vi "ZTarget.vi"(2 "PID gains for Z angle":T1={"proportional gain (Kc)"=0.03, "integral time (Ti, min)"=0.0, "derivative time (Td, min)"=0.001} {"derivative time (Td, min)" format="%.3f"; "integral time (Ti, min)" format="%.3f"; "proportional gain (Kc)" format="%.3f"}, 3 "Lower Array":dbl[](array[numeric])=[-14.0, 14.0, -59.0, 59.0, -121.0, 121.0, -166.0, 166.0, -180.0], 4 "Upper Array":dbl[](array[numeric])=[14.0, 59.0, -14.0, 121.0, -59.0, 166.0, -121.0, 190.0, -166.0], 5 "Target Values":dbl[](array[numeric])=[0.0, 28.0, -28.0, 90.0, -90.0, 152.0, -152.0, 180.0, 180.0], 6 "Zin":dbl) -> (0 "Z Out":dbl)   [LabVIEW 2018]
uses:
  Robot Global Data.vi
  <vilib>/addons/control/pid/pid.llb/PID (DBL).vi
  <vilib>/addons/control/pid/NI_PID_pid.lvlib
panel:
  out "ZTarget":dbl=180.0 format="%#_13g"
  out "In Range?":bool[](array[boolean])=[FALSE, FALSE, FALSE, FALSE, FALSE, FALSE, FALSE, FALSE, TRUE]
  in  "Auto Z":bool=TRUE
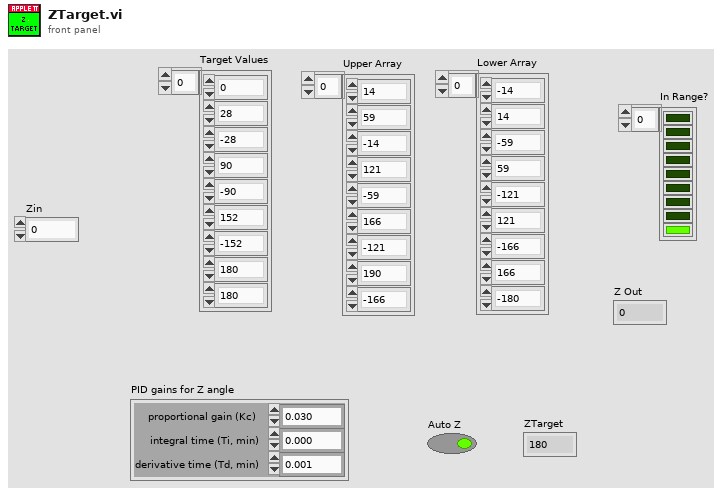
[diagram p1: front panel]
types:
  T1 = cluster{"proportional gain (Kc)":dbl, "integral time (Ti, min)":dbl, "derivative time (Td, min)":dbl}
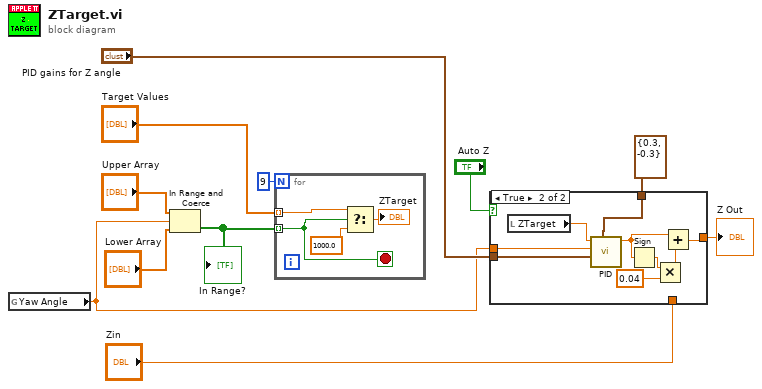
[diagram p0: block diagram]
diagram:
  n1 = global read "Robot Global Data.vi" "Yaw Angle"() -> (w3:dbl)
  n2 = In Range and Coerce(upper limit="Upper Array", x=w3, lower limit="Lower Array") -> (In Range?=w5:bool[])  [unwired: 1 out]
  "In Range?" <- w5
  n3 = for {
    N: 9 -> [_]
    tunnel: w5 -> [w12] mode=indexing
    tunnel: "Target Values" -> [w15] mode=indexing
    stop <- w12 stop-if-true
    n4 = Select(t=w15, s=w12, f=1000.0) -> (s? t:f=→"ZTarget":dbl)
  }
  n5 = case shown="True" "Auto Z" {
    tunnel: [w16 w19] -> w1
    tunnel: "PID gains for Z angle" -> [_ w25]
    tunnel: w3 -> [_ w24]
    tunnel: "Zin" -> [w16 _]
    tunnel: cluster{"output high":dbl, "output low":dbl} {"output high"=0.3, "output low"=-0.3} ("output range") -> [_ w17]
    frame False {
    }
    frame True {
      n6 = local read "ZTarget"() -> (w23:dbl)
      n7 = call-poly <vilib>:"PID.vi"("output range"=w17, "PID gains"=w25, "process variable"=w24, "setpoint"=w23) -> ("output"=w22:dbl)  [unwired: 6 in, 1 out]
      n8 = Sign(1:w22) -> (0:w21:dbl)
      n9 = Multiply(x=w21, y=0.04) -> (x*y=w18:dbl)
      n10 = Add(x=w22, y=w18) -> (x+y=w19:dbl)
    }
  }
  "Z Out" <- w1
